vi "StartLogging.vi"(8 "error in (no error)":errorcluster, 10 "Mode":T1 items=["Idle", "Snap", "Live", "Capturing", ""], 11 "DataLogger in":refnum<class "DataLogger.lvclass">) -> (0 "error out":errorcluster, 3 "DataLogger out":refnum<class "DataLogger.lvclass">)   [LabVIEW 2020, in "DataLogger.lvlib" / "DataLogger.lvclass"]
uses:
  DataLogger.lvclass
  C:/Program Files/National Instruments/LabVIEW 2020/vi.lib/ActorFramework/Actor/Actor.lvclass
  Hardware Layer/Real Hardware/Camera_Prime95B/Camera_Prime95B/Controls/Camera Status.ctl
  Hardware Layer/Real Hardware/Camera_Prime95B/Camera_Prime95B/Controls/AcquisitionParams.ctl
  Hardware Abstraction Layer/Component/Device/Device/DataExchange.ctl
  DataLogger.lvclass/DataLogger.ctl
  <vilib>/ActorFramework/Actor/Actor.lvclass/Actor.ctl
  Hardware Abstraction Layer/Component/Device/Device Messages/StartSequenceAcquisition Msg/StartSequenceAcquisition Msg.lvclass/StartSequenceAcquisition Msg.ctl
  <vilib>/ActorFramework/Message Enqueuer/Message Enqueuer.lvclass/Message Enqueuer.ctl
  <vilib>/ActorFramework/Message Enqueuer/Enqueue.vi
  Hardware Abstraction Layer/Component/Device/Device Messages/StartSequenceAcquisition Msg/StartSequenceAcquisition Msg.lvclass
  C:/Program Files/National Instruments/LabVIEW 2020/vi.lib/ActorFramework/Message/Message.lvclass
  <vilib>/ActorFramework/Message Priority Queue/Priority Enqueue.vi
  <vilib>/ActorFramework/Actor/Actor.lvclass
  Hardware Layer/Real Hardware/Camera_Prime95B/Camera_Prime95B/Camera_Prime95B.lvclass
  Interface/DataListener/DataListener.lvclass
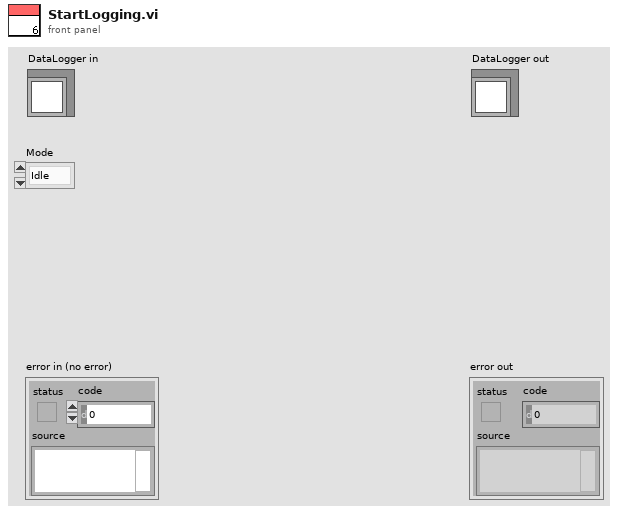
[diagram p1: front panel]
types:
  T1 = typedef "Camera_Prime95B.lvlib/Camera_Prime95B.lvclass/Camera Status.ctl" = i32
  T2 = typedef "DataListener.lvclass/DataExchange.ctl" = cluster{"Source":string, "Destination":string, "Description":string, "value":variant}
  T3 = typedef "Camera_Prime95B.lvlib/Camera_Prime95B.lvclass/AcquisitionParams.ctl" = cluster{"Acq Mode":T1, "Save Path":path, "Stream Save Path":path, "SingleStack?":bool, "StreamToDisk?":bool, "Alert when finish?":bool}
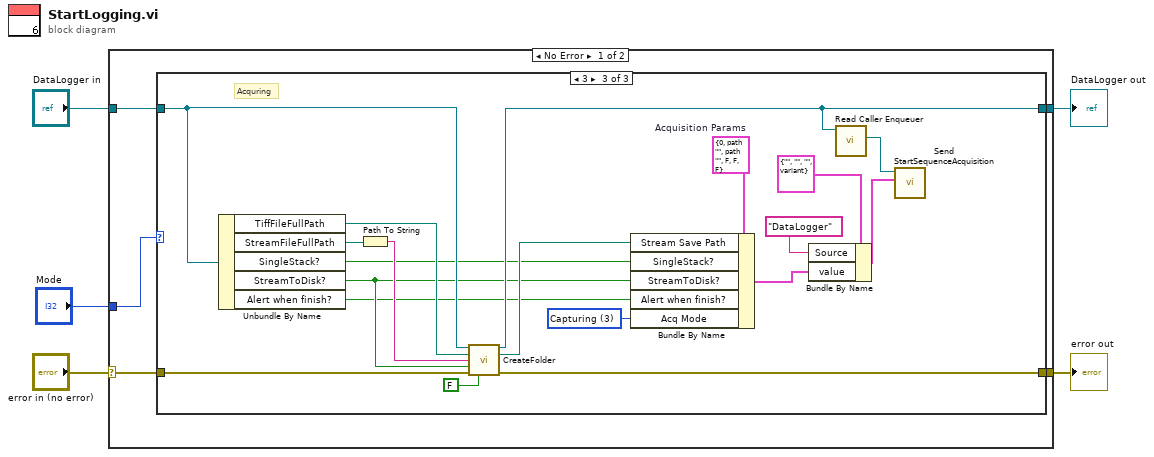
[diagram p0: block diagram]
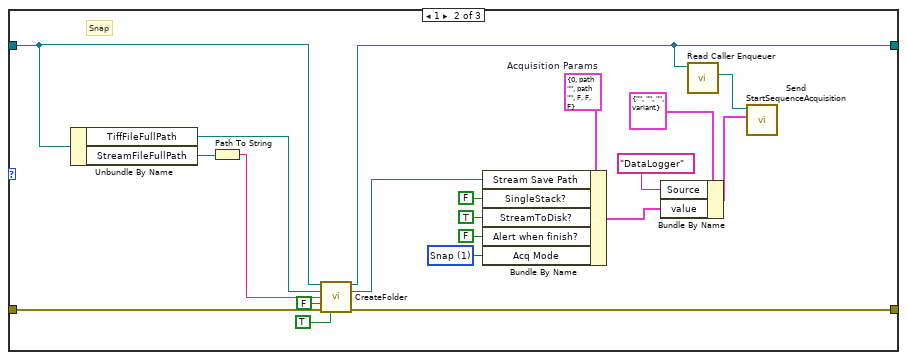
[diagram p3: hidden frame]
diagram:
  n1 = case shown="No Error" "error in (no error)" {
    selector: "error in (no error)" -> [w10 w53]
    tunnel: [w9 w53] -> w4
    tunnel: [w8 w52] -> w2
    tunnel: "DataLogger in" -> [w7 w52]
    tunnel: "Mode" -> [w6 _]
    frame No Error {
      n2 = case shown="3" w6 {
        tunnel: w10 -> [w11 w32 w51]
        tunnel: [w11 w31 w50] -> w9
        tunnel: [w12 w24 w43] -> w8
        tunnel: w7 -> [w12 w23 w42]
        frame 0, Default {
        }
        frame 1 {
          w13 = T1 1 items=["Idle", "Snap", "Live", "Capturing", ""] ("Acq Mode")
          w29 = T3 {"Acq Mode"=0, "Save Path"=path "", "Stream Save Path"=path "", "SingleStack?"=FALSE, "StreamToDisk?"=FALSE, "Alert when finish?"=FALSE}  # Acquisition Params
          # "Snap"
          n3 = Unbundle By Name(w23) -> ("TiffFileFullPath"=w22:path, "StreamFileFullPath"=w21:path)
          n4 = Path To String(path=w21) -> (string=w20:string)
          n5 = call-dynamic "CreateFolder.vi"("DataLogger in"=w23, "Save Path"=w22, "File suffix"=w20, "StreamToDisk?"=FALSE, "error in (no error)"=w32, "SnapShot?"=TRUE) -> ("DataLogger out"=w24:refnum<class "DataLogger.lvclass">, "Saving Path"=w17:path, "error out"=w31:errorcluster)  [unwired: 5 in, 2 out]
          n6 = Bundle By Name(cluster=w29, "Stream Save Path"=w17, "SingleStack?"=FALSE, "StreamToDisk?"=TRUE, "Alert when finish?"=FALSE, "Acq Mode"=w13) -> (w28:T3)
          n7 = Bundle By Name(cluster=T2 {"Source"="", "Destination"="", "Description"="", "value"=variant} ("input cluster"), "Source"="DataLogger", "value"=w28) -> (w26:T2)
          n8 = call <vilib>:"Read Caller Enqueuer.vi"("Actor"=w24) -> ("Caller Enqueuer"=w30:refnum<class "Message Enqueuer.lvclass">)  [unwired: 10 in]
          n9 = call "Send StartSequenceAcquisition.vi"("DataExchange"=w26, "Message Enqueuer"=w30) -> ()  [unwired: 8 in, 2 out]
        }
        frame 3 {
          w36 = T1 3 items=["Idle", "Snap", "Live", "Capturing", ""] ("Acq Mode")
          w48 = T3 {"Acq Mode"=0, "Save Path"=path "", "Stream Save Path"=path "", "SingleStack?"=FALSE, "StreamToDisk?"=FALSE, "Alert when finish?"=FALSE}  # Acquisition Params
          # "Acquring"
          n10 = Unbundle By Name(w42) -> ("TiffFileFullPath"=w41:path, "StreamFileFullPath"=w40:path, "SingleStack?"=w33:bool, "StreamToDisk?"=w35:bool, "Alert when finish?"=w34:bool)
          n11 = Path To String(path=w40) -> (string=w39:string)
          n12 = call-dynamic "CreateFolder.vi"("DataLogger in"=w42, "Save Path"=w41, "File suffix"=w39, "StreamToDisk?"=w35, "error in (no error)"=w51, "SnapShot?"=FALSE) -> ("DataLogger out"=w43:refnum<class "DataLogger.lvclass">, "Saving Path"=w37:path, "error out"=w50:errorcluster)  [unwired: 5 in, 2 out]
          n13 = Bundle By Name(cluster=w48, "Stream Save Path"=w37, "SingleStack?"=w33, "StreamToDisk?"=w35, "Alert when finish?"=w34, "Acq Mode"=w36) -> (w47:T3)
          n14 = Bundle By Name(cluster=T2 {"Source"="", "Destination"="", "Description"="", "value"=variant} ("input cluster"), "Source"="DataLogger", "value"=w47) -> (w45:T2)
          n15 = call <vilib>:"Read Caller Enqueuer.vi"("Actor"=w43) -> ("Caller Enqueuer"=w49:refnum<class "Message Enqueuer.lvclass">)  [unwired: 10 in]
          n16 = call "Send StartSequenceAcquisition.vi"("DataExchange"=w45, "Message Enqueuer"=w49) -> ()  [unwired: 8 in, 2 out]
        }
      }
    }
    frame Error {
    }
  }
  "error out" <- w4
  "DataLogger out" <- w2
